vi "禁用结构.vi"() -> ()   [LabVIEW 2010]
panel:
  out "运算结果":dbl
  in  "Y":dbl
  in  "X":dbl
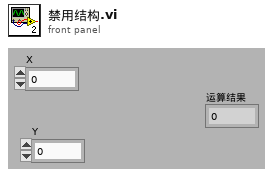
[diagram p1: front panel]
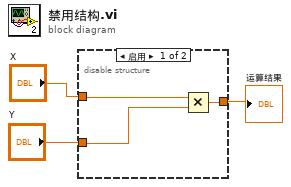
[diagram p0: block diagram]
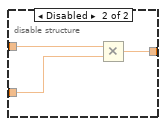
[diagram p2: hidden frame]
diagram:
  n1 = disable-structure shown="启用" {
    disable-tunnel: "X" -> [w6 w9]
    disable-tunnel: "Y" -> [w5 w8]
    disable-tunnel: [w4 w7] -> w1
    frame Enabled {
      n2 = Multiply(x=w6, y=w5) -> (x*y=w4:dbl)
    }
    frame Disabled {
      n3 = Multiply(x=w9, y=w8) -> (x*y=w7:dbl)
    }
  }
  "运算结果" <- w1
